vi "CalculateCaseStructureBorders.vi"(11 "Structure in":refnum<vi>) -> (3 "Structure border size":i32)   [LabVIEW 2017, in "ErrorStructureDrawer.lvlib"]
doc: "Calculates the border width for a case structure. Seems to be 6 pixels (for a default case structure at least - I'm not sure if it's possible to edit the border width?)"
uses:
  ErrorStructureDrawer.lvlib
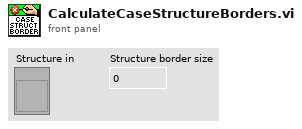
[diagram p1: front panel]
types:
  T1 = typedef "LVRectTypeDef.ctl" = cluster{"Left":i16, "Top":i16, "Right":i16, "Bottom":i16}
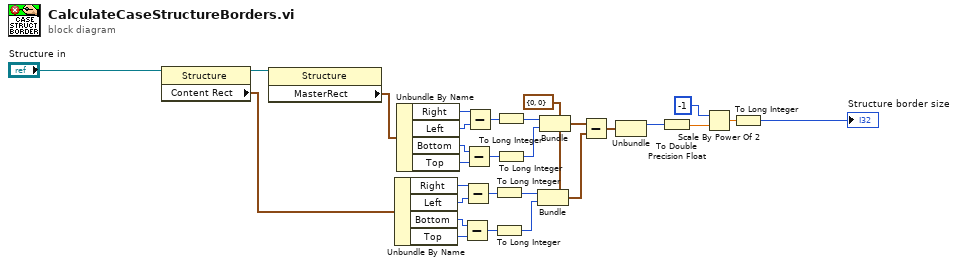
[diagram p0: block diagram]
diagram:
  w23 = cluster{"Width":i32, "Height":i32} {"Width"=0, "Height"=0} ("Dimensions")
  n1 = property class="Structure"(reference="Structure in") -> (reference out=w1:refnum<vi>, "Content Rect"=w20:T1)  [unwired: 1 in, 1 out]
  n2 = property class="Structure"(reference=w1) -> ("MasterRect"=w2:T1)  [unwired: 1 in, 2 out]
  n3 = Unbundle By Name(w20) -> ("Right"=w19:i16, "Left"=w18:i16, "Bottom"=w16:i16, "Top"=w17:i16)
  n4 = Unbundle By Name(w2) -> ("Right"=w3:i16, "Left"=w4:i16, "Bottom"=w6:i16, "Top"=w5:i16)
  n5 = Subtract(x=w16, y=w17) -> (x-y=w14:i16)
  n6 = Subtract(x=w19, y=w18) -> (x-y=w15:i16)
  n7 = Subtract(x=w6, y=w5) -> (x-y=w8:i16)
  n8 = Subtract(x=w3, y=w4) -> (x-y=w7:i16)
  n9 = To Long Integer(number=w15) -> (32bit integer=w13:i32)
  n10 = To Long Integer(number=w14) -> (32bit integer=w12:i32)
  n11 = To Long Integer(number=w7) -> (32bit integer=w9:i32)
  n12 = To Long Integer(number=w8) -> (32bit integer=w10:i32)
  n13 = Bundle(cluster=w23, "Width"=w13, "Height"=w12) -> (w21:cluster{"Width":i32, "Height":i32})
  n14 = Bundle(cluster=w23, "Width"=w9, "Height"=w10) -> (w11:cluster{"Width":i32, "Height":i32})
  n15 = Subtract(x=w11, y=w21) -> (x-y=w22:cluster{"Width":i32, "Height":i32})
  n16 = Unbundle(w22) -> ("Width"=w24:i32)  [unwired: 1 out]
  n17 = To Double Precision Float(number=w24) -> (double precision float=w25:dbl)
  n18 = Scale By Power Of 2(n=i16 -1, x=w25) -> (x*2^n=w27:dbl)
  n19 = To Long Integer(number=w27) -> (32bit integer=→"Structure border size":i32)
